vi "IT8800-Initialize.vi"(8 "error in (no error)":errorcluster, 11 "ITech Setting In":T1={"VISA Resource Name"="", "Baud Rate"=19200, "Stop Bits"=20, "Wait For Read(ms)"=0} {"Stop Bits" items=["1.0"=10, "2.0"=20]; "Baud Rate" items=["2400"=2400, "4800"=4800, "9600"=9600, "19200"=19200]}) -> (0 "error out":errorcluster, 3 "IT8800 Setting In Out":T1={"VISA Resource Name"="", "Baud Rate"=19200, "Stop Bits"=20, "Wait For Read(ms)"=0} {"Stop Bits" items=["1.0"=10, "2.0"=20]; "Baud Rate" items=["2400"=2400, "4800"=4800, "9600"=9600, "19200"=19200]})   [LabVIEW 2018]
doc: "Establishes communication with the instrument and optionally performs an instrument identification query and/or an instrument reset. It also places the instrument in a default state needed for other instrument driver operations. Therefore, call this VI before calling other instrument driver VIs for this instrument. Generally, you need to call the Initialize VI only once at the beginning of an application."
uses:
  Data Def/IT8800-Setting.ctl
  <vilib>/Instr/_visa.llb/VISA Configure Serial Port (Instr).vi
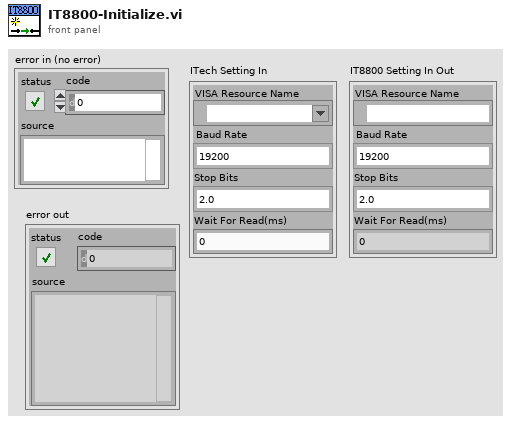
[diagram p1: front panel]
types:
  T1 = typedef "IT8800-Setting.ctl" = cluster{"VISA Resource Name":refnum<visa-resource-name>, "Baud Rate":u32, "Stop Bits":u16, "Wait For Read(ms)":u32}
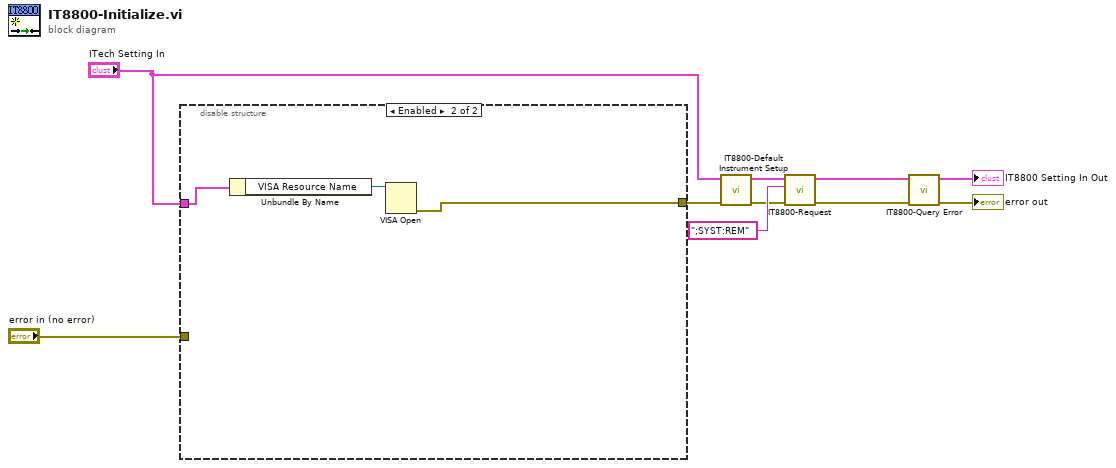
[diagram p0: block diagram]
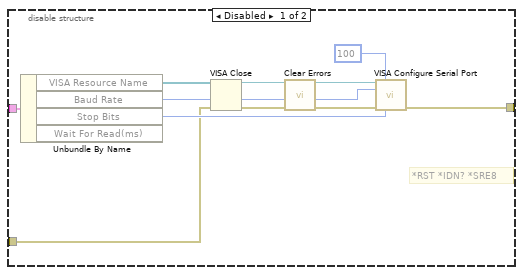
[diagram p2: hidden frame]
diagram:
  n1 = disable-structure shown="Enabled" {
    disable-tunnel: "error in (no error)" -> [w16 _]
    disable-tunnel: [w12 w20] -> w6
    disable-tunnel: "ITech Setting In" -> [w11 w22]
    frame Disabled {
      # "*RST *IDN? *SRE8"
      n2 = Unbundle By Name(w11) -> ("VISA Resource Name"=w15:refnum<visa-resource-name>, "Baud Rate"=w19:u32, "Stop Bits"=w18:u16)  [unwired: 1 out]
      n3 = VISA Close(VISA resource name=w15, error in (no error)=w16) -> (error out=w14:errorcluster)
      n4 = call <vilib>:"Clear Errors.vi"("error in (no error)"=w14) -> ("error out"=w13:errorcluster)  [unwired: 5 in, 1 out]
      n5 = call-poly "VISA Configure Serial Port"("VISA resource name"=w15, "timeout (10sec)"=u32 100, "baud rate (9600)"=w19, "error in (no error)"=w13, "stop bits (10: 1 bit)"=w18) -> ("error out"=w12:errorcluster)  [unwired: 9 in, 1 out]
    }
    frame Enabled {
      n6 = Unbundle By Name(w22) -> ("VISA Resource Name"=w21:refnum<visa-resource-name>)
      n7 = VISA Open(VISA resource name=w21) -> (error out=w20:errorcluster)  [unwired: 4 in, 1 out]
    }
  }
  n8 = call "IT8800-Default Instrument Setup.vi"("error in"=w6, "IT8800 Setting In In"="ITech Setting In") -> ("error out"=w5:errorcluster, "IT8800 Setting In Out"=w3:T1)  [unwired: 8 in]
  n9 = call "IT8800-Request.vi"("error in"=w5, "Command"=";SYST:REM" ("string"), "IT8800 Setting In In"=w3) -> ("error out"=w1:errorcluster, "IT8800 Setting In Out"=w2:T1)  [unwired: 6 in, 1 out]
  n10 = call "IT8800-Query Error.vi"("error in"=w1, "IT8800 Setting In In"=w2) -> ("error out"=→"error out":errorcluster, "IT8800 Setting In Out"=→"IT8800 Setting In Out":T1)  [unwired: 8 in]
